vi "751PotCalc_Resistance.vi"(0 "Vout":dbl, 2 "Vin":dbl, 3 "R1":dbl) -> (1 "Rx":dbl)   [LabVIEW 2025]
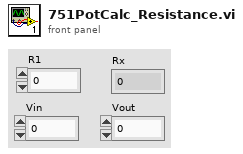
[diagram p1: front panel]
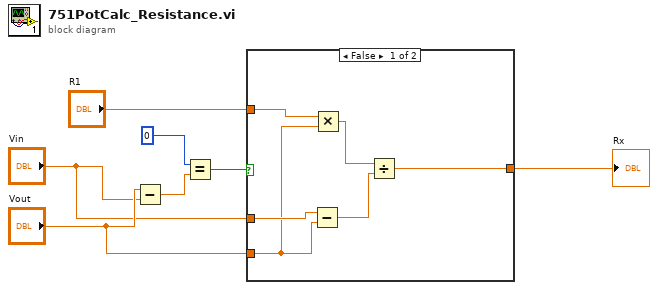
[diagram p0: block diagram]
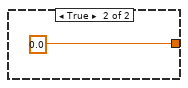
[diagram p2: hidden frame]
diagram:
  n1 = Subtract(x="Vout", y="Vin") -> (x-y=w6:dbl)
  n2 = Equal?(x=0, y=w6) -> (x = y?=w7:bool)
  n3 = case shown="False" w7 {
    tunnel: [w13 0.0] -> w1
    tunnel: "Vout" -> [w10 _]
    tunnel: "Vin" -> [w11 _]
    tunnel: "R1" -> [w12 _]
    frame False {
      n4 = Subtract(x=w11, y=w10) -> (x-y=w9:dbl)
      n5 = Multiply(x=w12, y=w10) -> (x*y=w8:dbl)
      n6 = Divide(x=w8, y=w9) -> (x/y=w13:dbl)
    }
    frame True {
    }
  }
  "Rx" <- w1
